vi "PumpInit.vi"() -> ()   [LabVIEW 2015]
panel:
  out "error out":errorcluster
  in  "Gearbox":dbl=4.75 format="%#_13g"
  in  "Stepper motor angle":dbl=1.8 format="%#_13g"
  in  "Backlash Correction":string
  in  "Volume Dispensed/pump rev":dbl=100.0 format="%#_13g"
  in  "Pump Address":string
  in  "Pump COMM Port":refnum<visa-resource-name>
  in  "error in (no error)":errorcluster
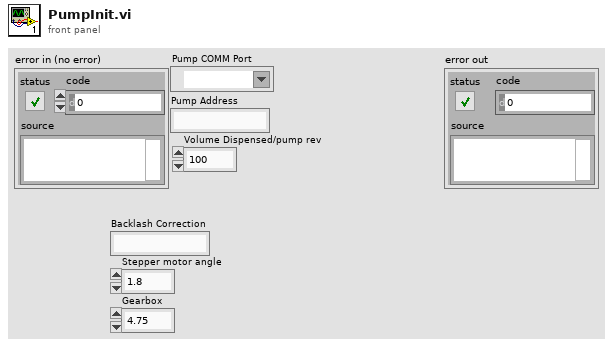
[diagram p1: front panel]
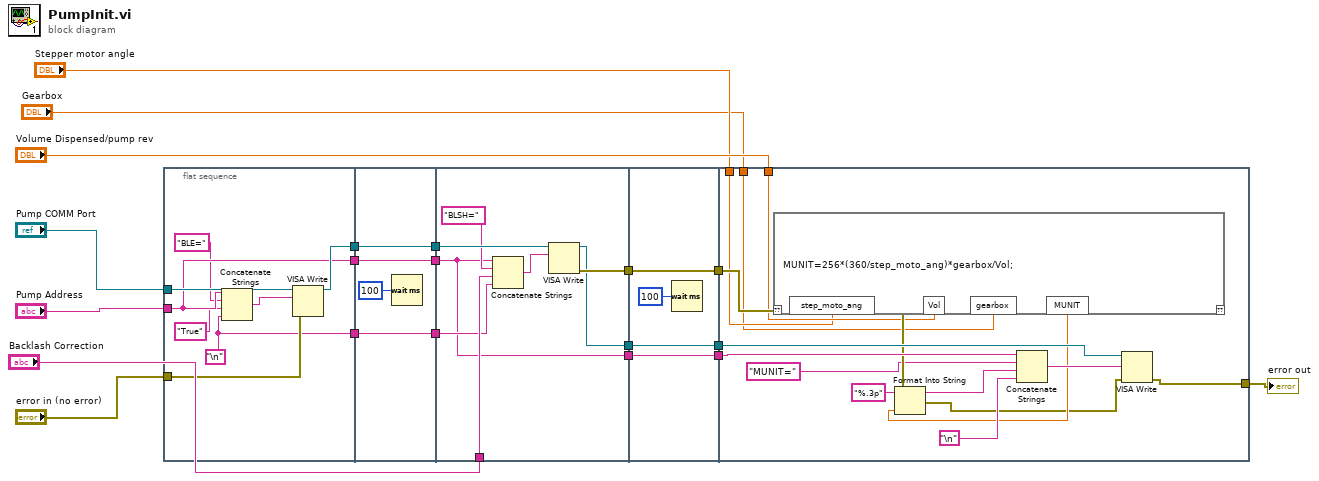
[diagram p0: block diagram]
diagram:
  n1 = flat-sequence {
    tunnel: "error in (no error)" -> [w27]
    tunnel: "Pump COMM Port" -> [w26]
    tunnel: [w25] -> w17
    tunnel: "Pump Address" -> [w24]
    tunnel: [w24] -> w14
    tunnel: [w23] -> w11
    tunnel: [w31] -> w18
    tunnel: w17 -> [w31]
    tunnel: [w30] -> w15
    tunnel: w14 -> [w30]
    tunnel: [w29] -> w12
    tunnel: w11 -> [w29]
    tunnel: w18 -> [w39]
    tunnel: w15 -> [w33]
    tunnel: "Backlash Correction" -> [w38]
    tunnel: w12 -> [w37]
    tunnel: [w35] -> w9
    tunnel: [w34] -> w7
    tunnel: [w33] -> w4
    tunnel: [w43] -> w10
    tunnel: w9 -> [w43]
    tunnel: [w42] -> w8
    tunnel: w7 -> [w42]
    tunnel: [w41] -> w5
    tunnel: w4 -> [w41]
    tunnel: w10 -> [w59]
    tunnel: w8 -> [w58]
    tunnel: [w57] -> w6
    tunnel: w5 -> [w53]
    tunnel: "Volume Dispensed/pump rev" -> [w47]
    tunnel: "Stepper motor angle" -> [w46]
    tunnel: "Gearbox" -> [w45]
    frame #0 {
      w23 = "\n"
      n2 = Concatenate Strings(w24, "BLE=" ("string"), "True" ("string"), w23) -> (w28:string)
      n3 = VISA Write(VISA resource name=w26, write buffer=w28, error in (no error)=w27) -> (VISA resource name out=w25:refnum<visa-resource-name>)  [unwired: 2 out]
    }
    frame #1 {
      n4 = Wait (ms)(milliseconds to wait=u32 100) -> ()  [unwired: 1 out]
    }
    frame #2 {
      n5 = Concatenate Strings(w33, "BLSH=" ("string"), w38, w37) -> (w40:string)
      n6 = VISA Write(VISA resource name=w39, write buffer=w40) -> (VISA resource name out=w34:refnum<visa-resource-name>, error out=w35:errorcluster)  [unwired: 1 in, 1 out]
    }
    frame #3 {
      n7 = Wait (ms)(milliseconds to wait=u32 100) -> ()  [unwired: 1 out]
    }
    frame #4 {
      n8 = script code="MUNIT=256*(360/step_moto_ang)*gearbox/Vol;"("??"=w59, "step_moto_ang"=w46, "Vol"=w47, "gearbox"=w45) -> ("??"=w49:errorcluster, "MUNIT"=w51:dbl)
      n9 = Format Into String(initial string="%.3p", error in=w49, w51) -> (resulting string=w54:string, error out=w50:errorcluster)  [unwired: 1 in]
      n10 = Concatenate Strings(w53, "MUNIT=" ("string"), w54, "\n") -> (w56:string)
      n11 = VISA Write(VISA resource name=w58, write buffer=w56, error in (no error)=w50) -> (error out=w57:errorcluster)  [unwired: 2 out]
    }
  }
  "error out" <- w6
